vi "TCP Read.vi"(8 "error in (no error)":errorcluster, 10 "timeout ms (1000)":i32=1000, 11 "Connection ID In":refnum<k5>) -> (0 "error out":errorcluster, 1 "Data Available?":bool, 2 "Read Data":string, 3 "Connection ID Out":refnum<k5>)   [LabVIEW 2016, in "SLL Easy API via TCP.lvclass"]
doc: "Check for any data available in TCP Buffer to Read. It expects the data if present, would have the string length at prefix/header of length 4 bytes."
uses:
  SLL Easy API via TCP.lvclass
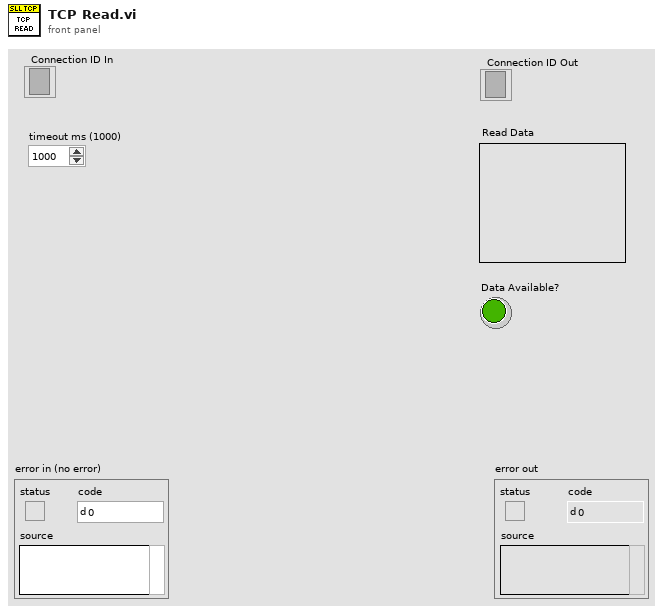
[diagram p1: front panel]
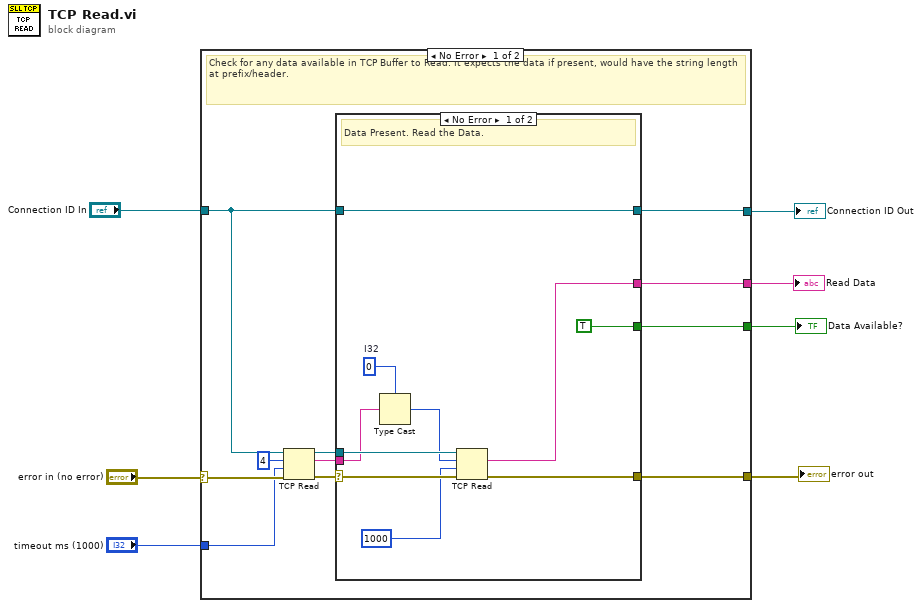
[diagram p0: block diagram]
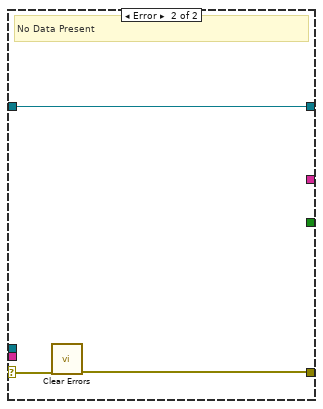
[diagram p2: hidden frame]
diagram:
  n1 = case shown="No Error" "error in (no error)" {
    selector: "error in (no error)" -> [w18 w33]
    tunnel: "Connection ID In" -> [w9 w32]
    tunnel: [w13 w33] -> w5
    tunnel: [w12 _] -> w4
    tunnel: [w11 _] -> w3
    tunnel: [w10 w32] -> w2
    tunnel: "timeout ms (1000)" -> [w8 _]
    frame No Error {
      # "Check for any data available in TCP Buffer to Read. It expects the data if present, would have the string length at prefix/header."
      n2 = TCP Read(connection ID=w9, bytes to read=4, error in (no error)=w18, 9:w8) -> (connection ID out=w15:refnum<k5>, data out=w14:string, error out=w16:errorcluster)  [unwired: 1 in]
      n3 = case shown="No Error" w16 {
        selector: w16 -> [w27 w31]
        tunnel: w15 -> [w28 _]
        tunnel: w14 -> [w26 _]
        tunnel: [w23 w30] -> w13
        tunnel: [w22 _] -> w12
        tunnel: [TRUE _] -> w11
        tunnel: [w20 w29] -> w10
        tunnel: w9 -> [w20 w29]
        frame No Error {
          w25 = 0  # I32
          # "Data Present. Read the Data."
          n4 = Type Cast(type=w25, x=w26) -> (*(type *) &x=w24:i32)
          n5 = TCP Read(connection ID=w28, bytes to read=w24, error in (no error)=w27, 9:1000 ("timeout ms (25000)")) -> (data out=w22:string, error out=w23:errorcluster)  [unwired: 1 in, 1 out]
        }
        frame Error {
          # "No Data Present"
          n6 = call <vilib>:"Clear Errors.vi"("error in (no error)"=w31) -> ("error out"=w30:errorcluster)  [unwired: 5 in, 1 out]
        }
      }
    }
    frame Error {
    }
  }
  "error out" <- w5
  "Data Available?" <- w3
  "Read Data" <- w4
  "Connection ID Out" <- w2
